vi "VsEPCal-Compute Sensitivity.vi"(0 "Atten (dB)":dbl[](array[numeric]), 1 "Params":T1, 5 "accelerometer (mV)":dbl[](array[numeric]), 11 "error in (no error)":errorcluster) -> (4 "Atten (dB) thru":dbl[](array[numeric]), 6 "accelerometer (mV) thru":dbl[](array[numeric]), 8 "Max Jerk (dB re 1g/ms)":dbl=-inf, 15 "error out":errorcluster)   [LabVIEW 2020]
uses:
  Typedefs/VsEPCal-Parameters.ctl
  Typedefs/VsEPCal- Stimulus.ctl
  Typedefs/VsEP-Hidden Params.ctl
  epl-vi-lib/Signal Synthesis VIs/Controls/Gate XCtl/Gate Control.xctl
  <vilib>/Analysis/baseanly.llb/Mean (DBL).vi
  epl-vi-lib/Utility VIs/Math VIs/Linear to dB (array).vi
  <vilib>/Analysis/NI_AALBase.lvlib
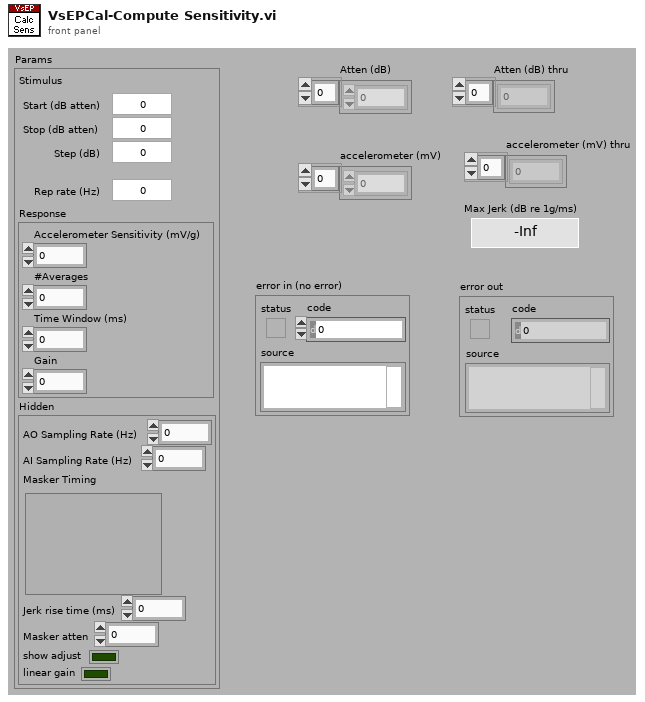
[diagram p1: front panel]
types:
  T1 = typedef "VsEPCal-Parameters.ctl" = cluster{"Stimulus":T2, "Response":cluster{"Accelerometer Sensitivity (mV/g)":dbl, "#Averages":i32, "Time Window (ms)":dbl, "Gain":dbl}, "Hidden":T3}
  T2 = typedef "VsEPCal- Stimulus.ctl" = cluster{"Rep rate (Hz)":dbl, "Start (dB atten)":dbl, "Stop (dB atten)":dbl, "Step (dB)":dbl}
  T3 = typedef "VsEP-Hidden Params.ctl" = cluster{"AO Sampling Rate (Hz)":dbl, "AI Sampling Rate (Hz)":dbl, "Masker Timing":cluster{"Active":bool, "Delay (ms)":dbl, "Width (ms)":dbl, "Ramp (ms)":dbl}, "Jerk rise time (ms)":dbl, "Masker atten":dbl, "show adjust":bool, "linear gain":bool}
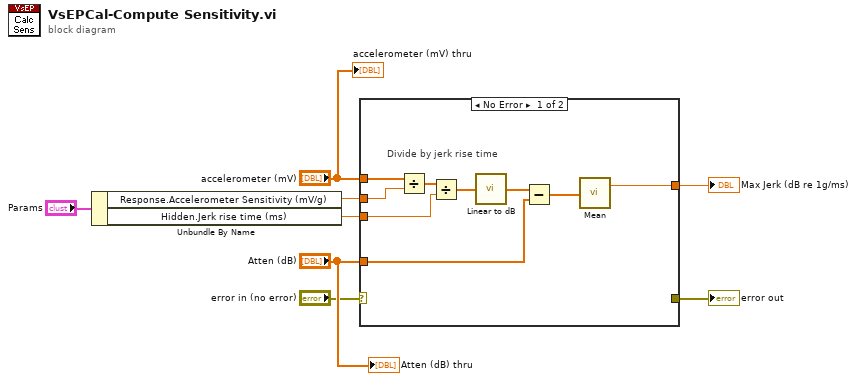
[diagram p0: block diagram]
diagram:
  n1 = Unbundle By Name("Params") -> ("Response.Accelerometer Sensitivity (mV/g)"=w2:dbl, "Hidden.Jerk rise time (ms)"=w1:dbl)
  n2 = case shown="No Error" "error in (no error)" {
    selector: "error in (no error)" -> [_ w18]
    tunnel: "accelerometer (mV)" -> [w16 _]
    tunnel: w2 -> [w15 _]
    tunnel: "Atten (dB)" -> [w12 _]
    tunnel: [w10 _] -> w6
    tunnel: [_ w18] -> w4
    tunnel: w1 -> [w9 _]
    frame No Error {
      # "Divide by jerk rise time"
      n3 = Divide(x=w16, y=w15) -> (x/y=w17:dbl[])
      n4 = Divide(x=w17, y=w9) -> (x/y=w14:dbl[])
      n5 = call-poly "Linear to dB.vi"("linear"=w14) -> ("dB"=w13:dbl[])
      n6 = Subtract(x=w13, y=w12) -> (x-y=w11:dbl[])
      n7 = call-poly <vilib>:"Mean.vi"("X"=w11) -> ("mean"=w10:dbl)  [unwired: 1 out]
    }
    frame Error {
    }
  }
  "error out" <- w4
  "Max Jerk (dB re 1g/ms)" <- w6
  "accelerometer (mV) thru" <- "accelerometer (mV)"
  "Atten (dB) thru" <- "Atten (dB)"
